vi "Opening VISA Devices.vi"(8 "에러 입력(에러 없음)":errorcluster, 11 "Device Ref In":T1 format="%.0x") -> (0 "에러 출력":errorcluster, 2 "VISA Outport":refnum<visa-resource-name>, 3 "VISA Inport":refnum<visa-resource-name>)   [LabVIEW 2017, in "Serial Communcation Devices Custom Device.lvlib"]
uses:
  Serial Communcation Devices Custom Device.lvlib
  <vilib>/NI Veristand/Custom Device API/Custom Device Item Ref.ctl
  <vilib>/Instr/_visa.llb/VISA Configure Serial Port (Instr).vi
  <vilib>/NI Veristand/Custom Device Tools/Custom Device Utility Library/Custom Device Utility Library.lvlib
  <vilib>/NI Veristand/Custom Device API/Custom Device API.lvlib
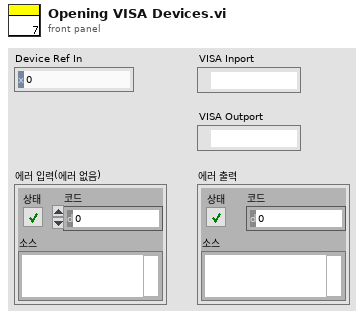
[diagram p1: front panel]
types:
  T1 = typedef "Custom Device API.lvlib/Custom Device Item Ref.ctl" = u64
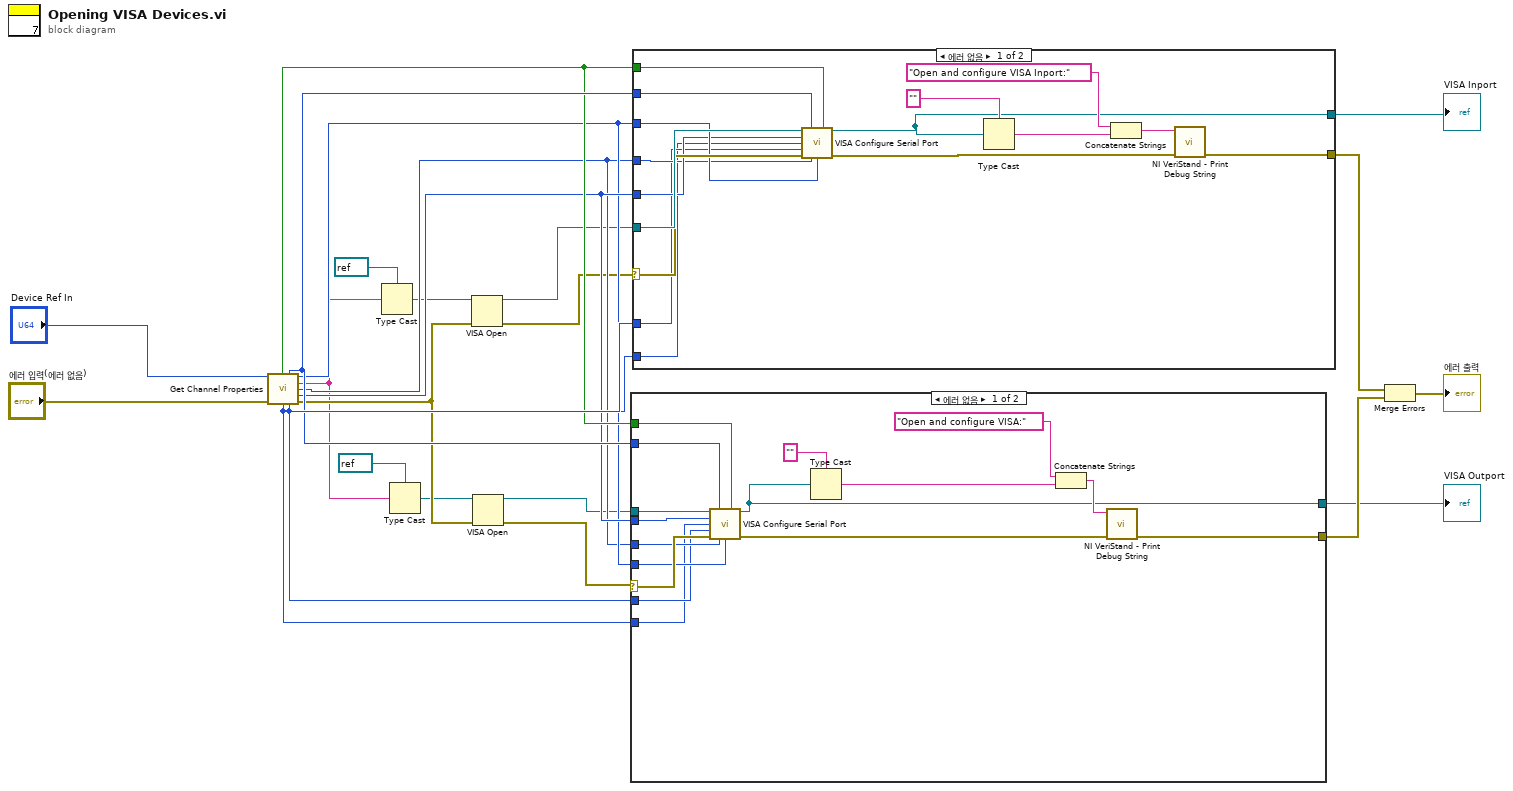
[diagram p0: block diagram]
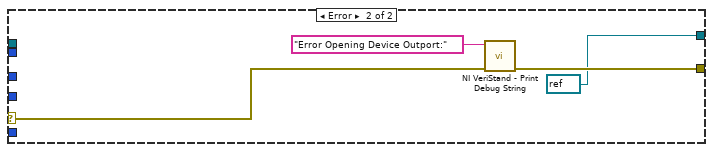
[diagram p2: hidden frame]
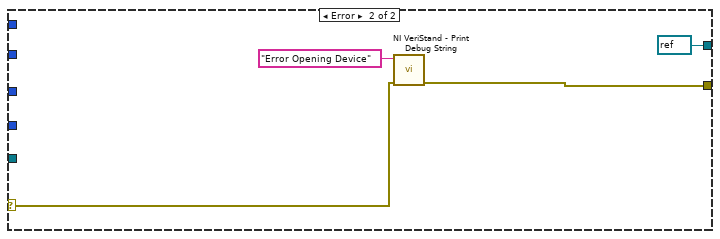
[diagram p3: hidden frame]
diagram:
  n1 = call "Get Channel Properties.vi"("Item Ref In"="Device Ref In", "에러 입력(에러 없음)"="에러 입력(에러 없음)") -> ("Enable Termination Char"=w18:bool, "Timeout"=w20:u16, "Flow Control"=w13:u16, "VISA\nResource\nName"=w10:string, "Stop Bits"=w12:u16, "Baud rate"=w15:u16, "Data bits"=w14:u16, "Parity"=w21:u16, "에러 출력"=w16:errorcluster)  [unwired: 4 in, 1 out]
  n2 = Type Cast(type=refnum<visa-resource-name> refnum ("VISA resource name"), x=w10) -> (*(type *) &x=w2:refnum<visa-resource-name>)
  n3 = Type Cast(type=refnum<visa-resource-name> refnum ("VISA resource name"), x=w10) -> (*(type *) &x=w8:refnum<visa-resource-name>)
  n4 = VISA Open(error in (no error)=w16, VISA resource name=w2) -> (VISA resource name=w3:refnum<visa-resource-name>, error out=w4:errorcluster)  [unwired: 3 in]
  n5 = VISA Open(error in (no error)=w16, VISA resource name=w8) -> (VISA resource name=w11:refnum<visa-resource-name>, error out=w17:errorcluster)  [unwired: 3 in]
  n6 = case shown="에러 없음" w17 {
    selector: w17 -> [w39 w44]
    tunnel: w11 -> [w40 _]
    tunnel: [w37 w43] -> w23
    tunnel: [w32 refnum<visa-resource-name> refnum ("VISA resource name")] -> w19
    tunnel: w13 -> [w31 _]
    tunnel: w15 -> [w30 _]
    tunnel: w12 -> [w29 _]
    tunnel: w18 -> [w28 _]
    tunnel: w20 -> [w27 _]
    tunnel: w21 -> [w26 _]
    tunnel: w14 -> [w25 _]
    frame No Error {
      n7 = call-poly "VISA Configure Serial Port"("VISA resource name"=w40, "timeout (10sec)"=w27, "Enable Termination\nChar (T)"=w28, "baud rate (9600)"=w30, "data bits (8)"=w25, "parity (0:none)"=w26, "error in (no error)"=w39, "stop bits (10: 1 bit)"=w29, "flow control (0:none)"=w31) -> ("VISA resource name out"=w32:refnum<visa-resource-name>, "error out"=w38:errorcluster)  [unwired: 5 in]
      n8 = Type Cast(type="", x=w32) -> (*(type *) &x=w33:string)
      n9 = Concatenate Strings("Open and configure VISA:", w33) -> (w34:string)
      n10 = call "NI VeriStand - Print Debug String.vi"("error in (no error)"=w38, "Message"=w34) -> ("error out"=w37:errorcluster)  [unwired: 9 in]
    }
    frame Error {
      n11 = call "NI VeriStand - Print Debug String.vi"("error in (no error)"=w44, "Message"="Error Opening Device Outport:") -> ("error out"=w43:errorcluster)  [unwired: 9 in]
    }
  }
  "VISA Outport" <- w19
  n12 = case shown="에러 없음" w4 {
    selector: w4 -> [w59 w64]
    tunnel: w3 -> [w60 _]
    tunnel: [w57 w63] -> w22
    tunnel: [w52 refnum<visa-resource-name> refnum ("VISA resource name")] -> w7
    tunnel: w13 -> [w51 _]
    tunnel: w15 -> [w50 _]
    tunnel: w12 -> [w49 _]
    tunnel: w18 -> [w48 _]
    tunnel: w20 -> [w47 _]
    tunnel: w21 -> [w46 _]
    tunnel: w14 -> [w45 _]
    frame No Error {
      n13 = call-poly "VISA Configure Serial Port"("VISA resource name"=w60, "timeout (10sec)"=w47, "Enable Termination\nChar (T)"=w48, "baud rate (9600)"=w50, "data bits (8)"=w45, "parity (0:none)"=w46, "error in (no error)"=w59, "stop bits (10: 1 bit)"=w49, "flow control (0:none)"=w51) -> ("VISA resource name out"=w52:refnum<visa-resource-name>, "error out"=w58:errorcluster)  [unwired: 5 in]
      n14 = Type Cast(type="", x=w52) -> (*(type *) &x=w53:string)
      n15 = Concatenate Strings("Open and configure VISA Inport:", w53) -> (w54:string)
      n16 = call "NI VeriStand - Print Debug String.vi"("error in (no error)"=w58, "Message"=w54) -> ("error out"=w57:errorcluster)  [unwired: 9 in]
    }
    frame Error {
      n17 = call "NI VeriStand - Print Debug String.vi"("error in (no error)"=w64, "Message"="Error Opening Device") -> ("error out"=w63:errorcluster)  [unwired: 9 in]
    }
  }
  "VISA Inport" <- w7
  n18 = Merge Errors(w22, w23) -> (→"에러 출력":errorcluster)
